vi "tearDown.vi"(8 "error in (no error)":errorcluster, 11 "reference in":refnum<class "Instrument Addon Scripting API Messages Unit Tests.lvclass">) -> (0 "error out":errorcluster, 3 "reference out":refnum<class "Instrument Addon Scripting API Messages Unit Tests.lvclass">)   [LabVIEW 2019, in "Instrument Addon Scripting API Messages Unit Tests.lvclass"]
doc: "tearDown runs after the test method has completed. Use this method to clean up any operations or references that were opened by setUp or the test method. Unit tests should be independent of other unit tests so this VI should ensure that the next test can run in a 'clean' test environment."
uses:
  Instrument Addon Scripting API Messages Unit Tests.lvclass
  Instrument Addon Scripting API Messages Unit Tests.lvclass/Instrument Addon Scripting API Messages Unit Tests.ctl
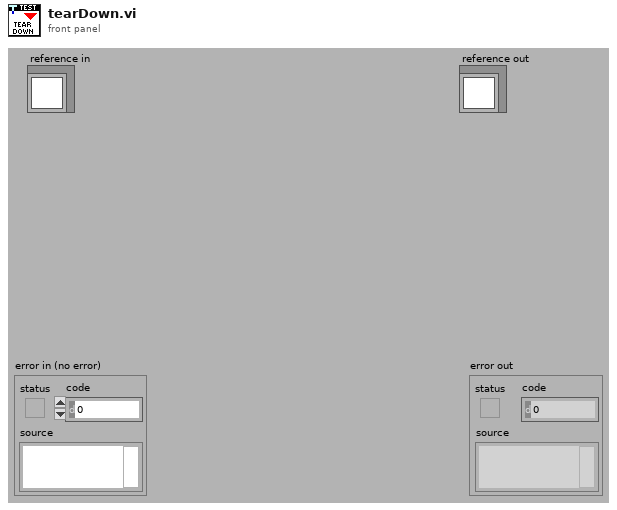
[diagram p1: front panel]
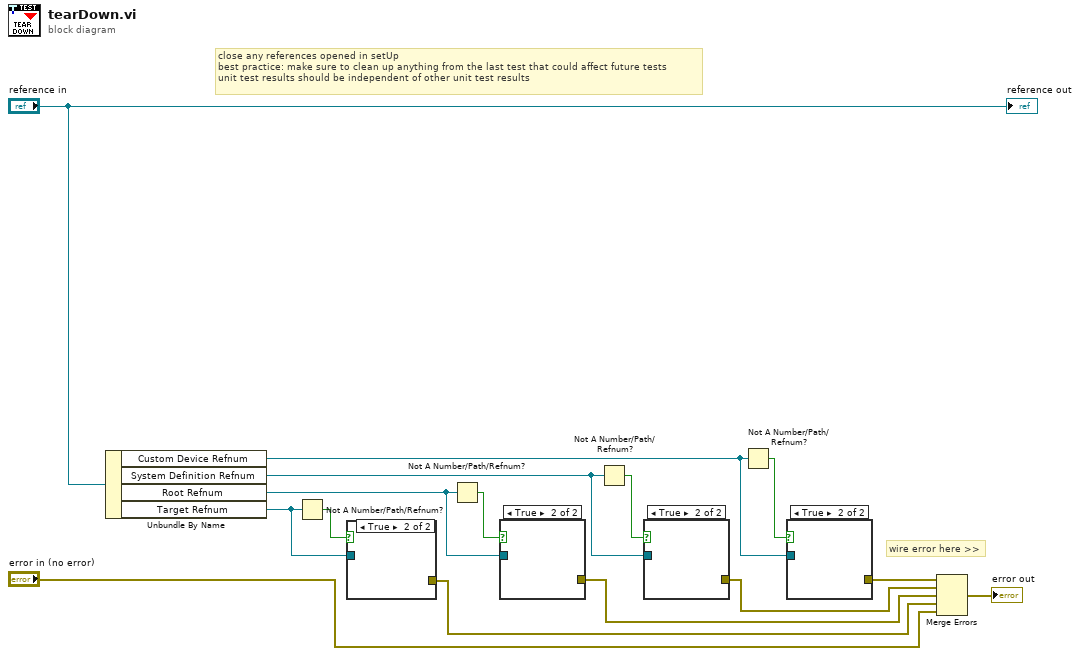
[diagram p0: block diagram]
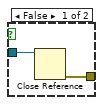
[diagram p2: hidden frame]
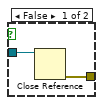
[diagram p3: hidden frame]
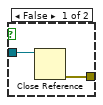
[diagram p4: hidden frame]
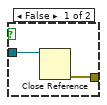
[diagram p5: hidden frame]
diagram:
  # "wire error here >>"
  # "close any references opened in setUp\nbest practice: make sure to clean up anything from the last test that could affect future tests\nunit test results should be independent of other unit test results"
  n1 = Unbundle By Name("reference in") -> ("Custom Device Refnum"=w3:refnum<k24>, "System Definition Refnum"=w10:refnum<k24>, "Root Refnum"=w12:refnum<k24>, "Target Refnum"=w14:refnum<k24>)
  n2 = Not A Number/Path/Refnum?(number/path/refnum=w14) -> (NaN/Path/Refnum?=w15:bool)
  n3 = case shown="True" w15 {
    tunnel: w14 -> [w17 _]
    tunnel: [w16 _] -> w7
    frame False {
      n4 = Close Reference(reference=w17) -> (error out=w16:errorcluster)  [unwired: 1 in]
    }
    frame True {
    }
  }
  n5 = Not A Number/Path/Refnum?(number/path/refnum=w12) -> (NaN/Path/Refnum?=w13:bool)
  n6 = case shown="True" w13 {
    tunnel: w12 -> [w19 _]
    tunnel: [w18 _] -> w8
    frame False {
      n7 = Close Reference(reference=w19) -> (error out=w18:errorcluster)  [unwired: 1 in]
    }
    frame True {
    }
  }
  n8 = Not A Number/Path/Refnum?(number/path/refnum=w10) -> (NaN/Path/Refnum?=w11:bool)
  n9 = case shown="True" w11 {
    tunnel: w10 -> [w21 _]
    tunnel: [w20 _] -> w9
    frame False {
      n10 = Close Reference(reference=w21) -> (error out=w20:errorcluster)  [unwired: 1 in]
    }
    frame True {
    }
  }
  n11 = Not A Number/Path/Refnum?(number/path/refnum=w3) -> (NaN/Path/Refnum?=w4:bool)
  n12 = case shown="True" w4 {
    tunnel: w3 -> [w23 _]
    tunnel: [w22 _] -> w2
    frame False {
      n13 = Close Reference(reference=w23) -> (error out=w22:errorcluster)  [unwired: 1 in]
    }
    frame True {
    }
  }
  n14 = Merge Errors(w2, w9, w8, w7, "error in (no error)") -> (→"error out":errorcluster)
  "reference out" <- "reference in"
